vi "Write Threshold.vi"(8 "error in (no error)":errorcluster, 10 "Threshold":dbl, 11 "ThresholdProcessor1D in":refnum<class "ThresholdProcessor1D.lvclass">) -> (0 "error out":errorcluster, 3 "ThresholdProcessor1D out":refnum<class "ThresholdProcessor1D.lvclass">)   [LabVIEW 2014, in "ThresholdProcessor1D.lvclass"]
uses:
  ThresholdProcessor1D.lvclass
  ThresholdProcessor1D.lvclass/ThresholdProcessor1D.ctl
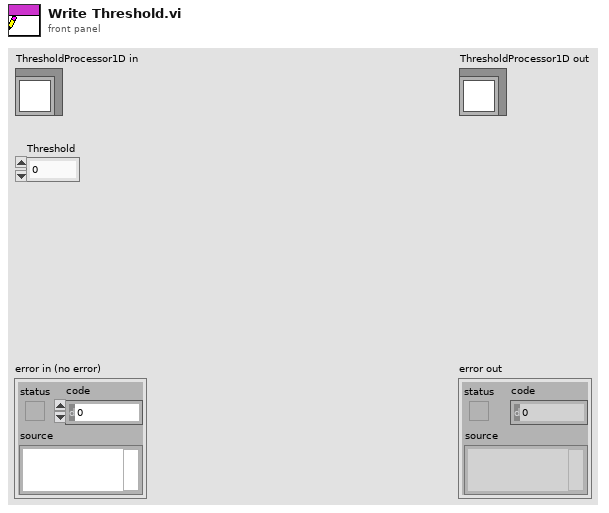
[diagram p1: front panel]
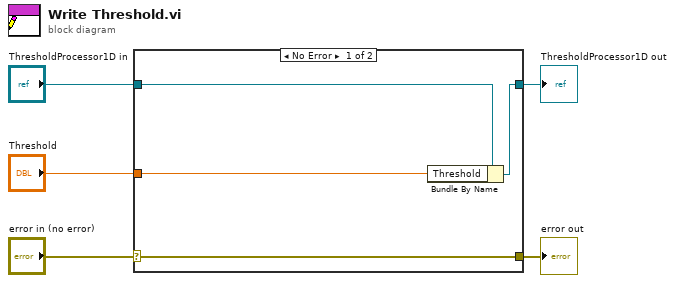
[diagram p0: block diagram]
diagram:
  n1 = case shown="No Error" "error in (no error)" {
    selector: "error in (no error)" -> [w9 w10]
    tunnel: [w9 w10] -> w4
    tunnel: [w7 w11] -> w2
    tunnel: "ThresholdProcessor1D in" -> [w8 w11]
    tunnel: "Threshold" -> [w6 _]
    frame No Error {
      n2 = Bundle By Name(cluster=w8, "Threshold"=w6) -> (w7:refnum<class "ThresholdProcessor1D.lvclass">)
    }
    frame Error {
    }
  }
  "error out" <- w4
  "ThresholdProcessor1D out" <- w2
